vi "jMsg_TCPClient_Connection_Update - Rx Read.vi"(8 "error in (no error)":errorcluster, 11 "jModule":refnum<class "jModule.lvclass">) -> (0 "error out":errorcluster, 1 "IP Address":string, 2 "Port":u16, 3 "jModule":refnum<class "jModule.lvclass">, 7 "jMsg_TCPClient_Connection_Update":refnum<class "jMsg_TCPClient_Connection_Update.lvclass">)   [LabVIEW 2019, in "jMsg_TCPClient_Connection_Update.lvclass"]
doc: "This VI is used to read data from the jMsg\n\n\nJSMA Message Wizard 0.2.0.5\nRob Humfeld - Jet Engineering\nCopyright (c) 2020, Jet Engineering"
uses:
  jMsg_TCPClient_Connection_Update.lvclass
  <userlib>/Jet Engineering/JSMA/Libraries/jModule Class/jModule.lvclass
  <userlib>/Jet Engineering/JSMA/Libraries/jModule Class/jModule.lvclass/jModule.ctl
  jMsg_TCPClient_Connection_Update.lvclass/jMsg_TCPClient_Connection_Update.ctl
panel:
  in  "jMsg_TCPClient_Connection_Update":refnum<class "jMsg_TCPClient_Connection_Update.lvclass">
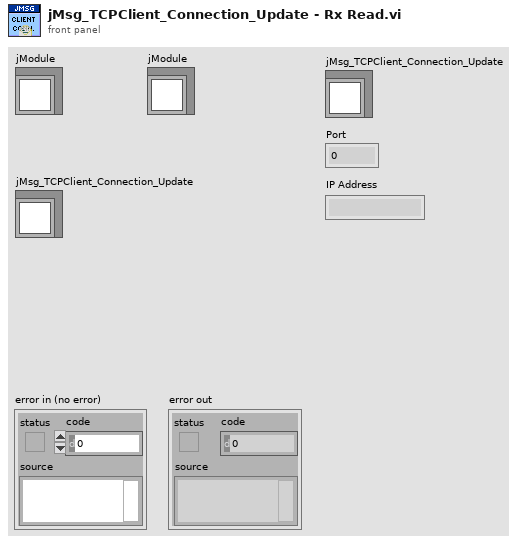
[diagram p1: front panel]
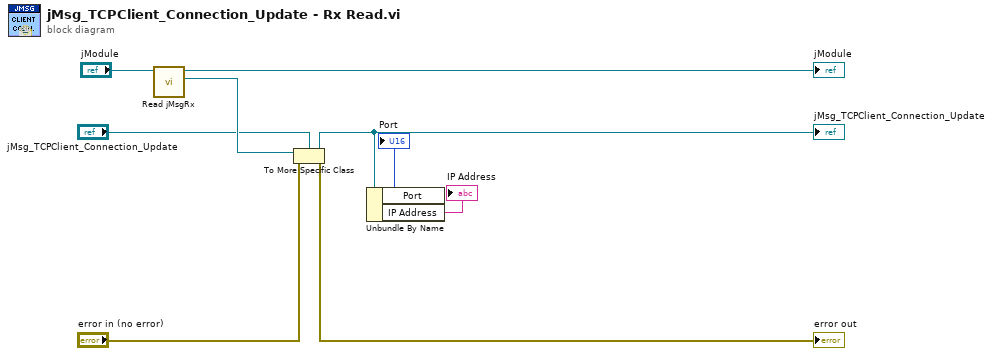
[diagram p0: block diagram]
diagram:
  n1 = call <userlib>:"Read jMsgRx.vi"("jModule in"="jModule") -> ("Received jMsg"=w6:refnum<class "jMsg.lvclass">, "jModule out"=→"jModule":refnum<class "jModule.lvclass">)  [unwired: 8 in, 1 out]
  n2 = To More Specific Class(target class="jMsg_TCPClient_Connection_Update", reference=w6, error in="error in (no error)") -> (specific class reference=w9:refnum<class "jMsg_TCPClient_Connection_Update.lvclass">, error out=→"error out":errorcluster)
  "jMsg_TCPClient_Connection_Update" <- w9
  n3 = Unbundle By Name(w9) -> ("Port"=→"Port":u16, "IP Address"=→"IP Address":string)
